vi "Write Gui_Configurating.vi"(8 "error in (no error)":errorcluster, 10 "Gui_Configurating":T1, 11 "GUI_Handler_Main in":refnum<class "GUI_Handler_Main.lvclass">) -> (0 "error out":errorcluster, 3 "GUI_Handler_Main out":refnum<class "GUI_Handler_Main.lvclass">)   [LabVIEW 2017, in "GUI_Handler_Main.lvclass"]
uses:
  GUI_Handler_Main.lvclass
  GUI_Handler_Main.lvclass/GUI_Handler_Main.ctl
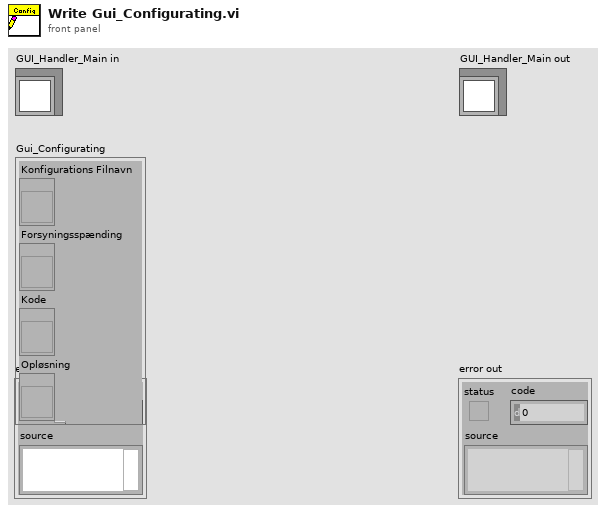
[diagram p1: front panel]
types:
  T1 = cluster{"Konfigurations Filnavn":refnum<vi>, "Forsyningsspænding":refnum<vi>, "Kode":refnum<vi>, "Opløsning":refnum<vi>}
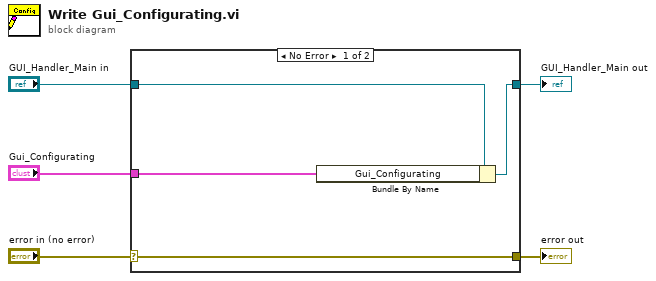
[diagram p0: block diagram]
diagram:
  n1 = case shown="No Error" "error in (no error)" {
    selector: "error in (no error)" -> [w9 w10]
    tunnel: [w9 w10] -> w4
    tunnel: [w7 w11] -> w2
    tunnel: "GUI_Handler_Main in" -> [w8 w11]
    tunnel: "Gui_Configurating" -> [w6 _]
    frame No Error {
      n2 = Bundle By Name(cluster=w8, "Gui_Configurating"=w6) -> (w7:refnum<class "GUI_Handler_Main.lvclass">)
    }
    frame Error {
    }
  }
  "error out" <- w4
  "GUI_Handler_Main out" <- w2
